vi "Pre Launch Init.vi"(11 "ResultsViewer in":refnum<class "ResultsViewer.lvclass">) -> (0 "error out":errorcluster, 3 "ResultsViewer out":refnum<class "ResultsViewer.lvclass">)   [LabVIEW 2019, in "ResultsViewer.lvlib" / "ResultsViewer.lvclass"]
doc: "(<B>Filename</B>: Actor Framework.lvlib:Actor.lvclass:Pre Launch Init.vi)\n\nDefines behavior that occurs after the Launch Nested Actor method is invoked but before the actor's Actor Core method begins running.\n\nBy default, this method does nothing. A descendant class may override it to define behavior."
uses:
  ResultsViewer.lvclass
  ResultsViewer.lvclass/ResultsViewer.ctl
  <vilib>/ActorFramework/Actor/Actor.lvclass
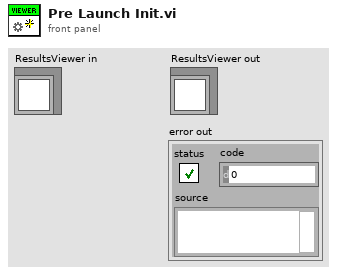
[diagram p1: front panel]
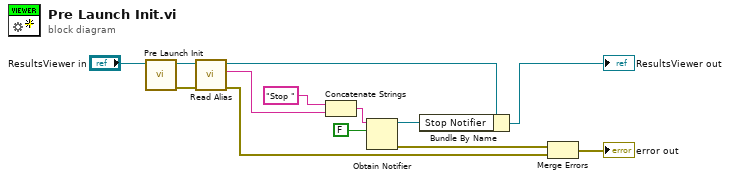
[diagram p0: block diagram]
diagram:
  n1 = call-parent "Pre Launch Init.vi"("Actor in"="ResultsViewer in") -> ("error out"=w13:errorcluster, "Actor out"=w5:refnum<class "ResultsViewer.lvclass">)  [unwired: 9 in]
  n2 = call-dynamic "Read Alias.vi"("error in (no error)"=w13, "ResultsViewer in"=w5) -> ("error out"=w6:errorcluster, "Alias"=w3:string, "ResultsViewer out"=w4:refnum<class "ResultsViewer.lvclass">)  [unwired: 7 in]
  n3 = Concatenate Strings("Stop " ("string"), w3) -> (w2:string)
  n4 = Obtain Notifier(name (unnamed)=w2, notification data type=FALSE) -> (notifier out=w8:refnum<notifier>, error out=w7:errorcluster)  [unwired: 2 in, 1 out]
  n5 = Bundle By Name(cluster=w4, "Stop Notifier"=w8) -> (→"ResultsViewer out":refnum<class "ResultsViewer.lvclass">)
  n6 = Merge Errors(w7, w6) -> (→"error out":errorcluster)
